vi "CLC_Gen3_L2_Manual_GUI.vi"() -> ()   [LabVIEW 2023, in "Clover_Cell.lvlib"]
uses:
  Clover_Cell.lvlib
  lib/Anritsu Signal Analyzer Series/Anritsu Signal Analyzer Series.lvlib
panel:
  in  "clear":bool
  out "Waveform Chart":dbl(graph)
  in  "Close":bool
  out "AvgTimes 2":i32=3
  out "Looping Times":i32
  out "error out":errorcluster
  in  "AvgTimes":i32=3
  in  "Start":bool
  in  "stop":bool
  in  "CenterFreq(GHz)":dbl=28.0
  in  "VISA resource name":refnum<visa-resource-name>="TCPIP0::192.168.100.230::inst0::INSTR"
  # "SA Record Tool ( Only )"
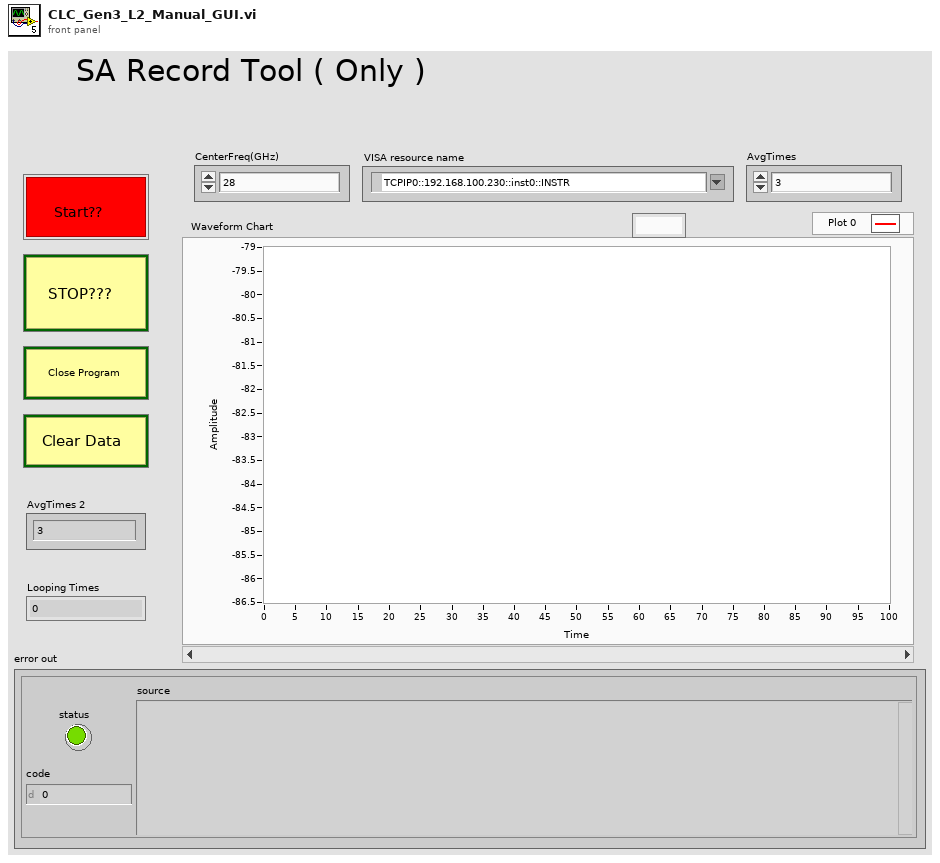
[diagram p1: front panel]
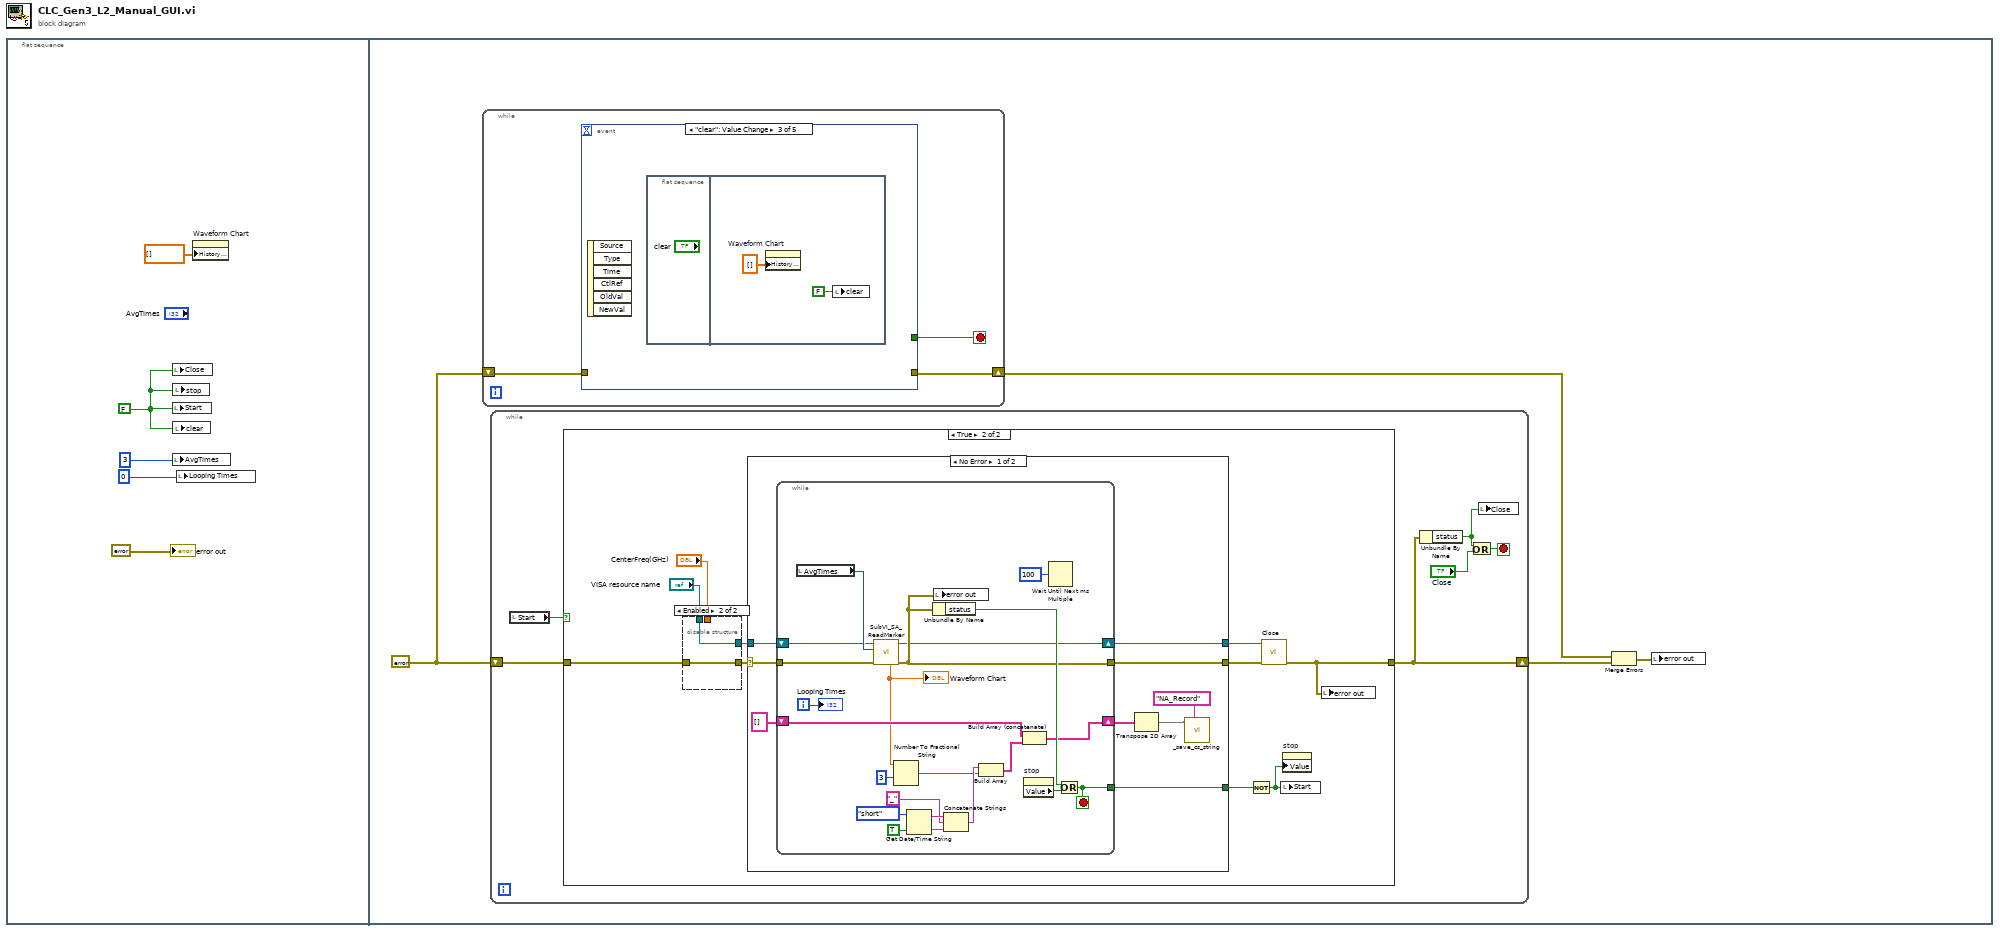
[diagram p0: block diagram]
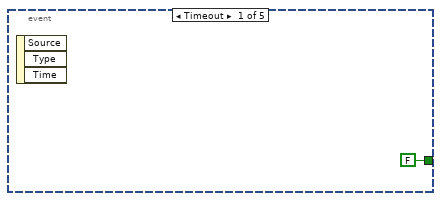
[diagram p2: hidden frame]
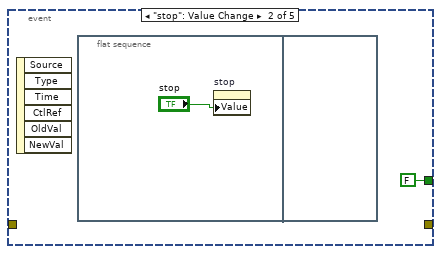
[diagram p3: hidden frame]
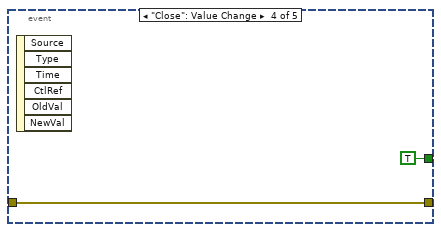
[diagram p4: hidden frame]
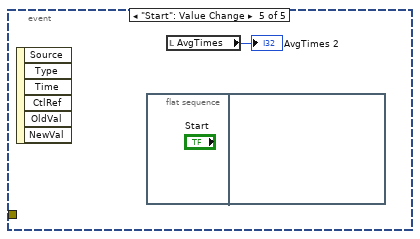
[diagram p5: hidden frame]
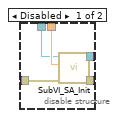
[diagram p7: hidden frame]
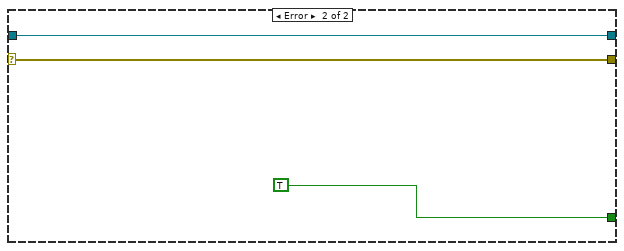
[diagram p8: hidden frame]
diagram:
  n1 = flat-sequence {
    frame #0 {
      w1 = FALSE ("Initialize")
      n2 = local write "Close"(w1) -> ()
      n3 = local write "Start"(w1) -> ()
      n4 = local write "AvgTimes"(3 ("AvgTimes")) -> ()
      n5 = local write "stop"(w1) -> ()
      n6 = local write "clear"(w1) -> ()
      n7 = local write "Looping Times"(0 ("Looping Times")) -> ()
      n8 = property on="Waveform Chart" class="WFChart (strict)"("History Data"=dbl[] []) -> ()  [unwired: 2 in, 2 out]
      "error out" <- errorcluster {"status"=FALSE, "code"=0, "source"=""} ("error in (no error)")
    }
    frame #1 {
      w9 = errorcluster {"status"=FALSE, "code"=0, "source"=""} ("error in (no error)")
      n9 = while {
        shift-right: [w10] -> w8
        shift-left: w9 -> [w11]
        stop <- w12 stop-if-true
        n10 = event shown="[2] \"clear\": Value Change" {
          selector: _ -> [_ _ _ _ _]
          dyn-events: _ -> [_ _ _ _ _]
          timeout: _ -> [_ _ _ _ _]
          tunnel: [FALSE ("stop") FALSE ("stop") _ TRUE ("stop") _] -> w12
          tunnel: w11 -> [_ _ _ w18 _]
          tunnel: [_ _ _ w18 _] -> w10
          event Timeout {
            n11 = event-data() -> ()  [unwired: 1 in, 3 out]
          }
          event "stop": Value Change {
            n12 = event-data() -> ()  [unwired: 1 in, 6 out]
            n13 = flat-sequence {
              frame #0 {
                n14 = property on="stop" class="Bool (strict)"("Value"="stop") -> ()  [unwired: 2 in, 2 out]
              }
              frame #1 {
              }
            }
          }
          event "clear": Value Change {
            n15 = event-data() -> ()  [unwired: 1 in, 6 out]
            n16 = flat-sequence {
              frame #0 {
              }
              frame #1 {
                n17 = property on="Waveform Chart" class="WFChart (strict)"("History Data"=dbl[] []) -> ()  [unwired: 2 in, 2 out]
                n18 = local write "clear"(FALSE ("clear")) -> ()
              }
            }
          }
          event "Close": Value Change {
            n19 = event-data() -> ()  [unwired: 1 in, 6 out]
          }
          event "Start": Value Change {
            n20 = event-data() -> ()  [unwired: 1 in, 6 out]
            n21 = flat-sequence {
              frame #0 {
              }
              frame #1 {
              }
            }
            n22 = local read "AvgTimes"() -> (→"AvgTimes 2":i32)
          }
        }
      }
      n23 = while {
        shift-right: [w24] -> w7
        shift-left: w9 -> [w25]
        stop <- w22 stop-if-true
        n24 = local read "Start"() -> (w26:bool)
        n25 = case shown="True" w26 {
          tunnel: w25 -> [w27 w31]
          tunnel: [w27 w33] -> w24
          frame False {
          }
          frame True {
            n26 = disable-structure shown="Enabled" {
              disable-tunnel: "CenterFreq(GHz)" -> [w42 _]
              disable-tunnel: w31 -> [w41 w44]
              disable-tunnel: "VISA resource name" -> [w40 w43]
              disable-tunnel: [w39 w43] -> w29
              disable-tunnel: [w38 w44] -> w28
              frame Disabled {
                n27 = call "SubVI_SA_Init.vi"("error in (no error)"=w41, "CenterFreq(GHz) 2"=w42, "VISA resource name"=w40) -> ("error out 2"=w38:errorcluster, "VISA resource name out"=w39:refnum<visa-resource-name>)  [unwired: 6 in, 1 out]
              }
              frame Enabled {
              }
            }
            n28 = case shown="No Error" w28 {
              selector: w28 -> [w49 w78]
              tunnel: [w53 TRUE] -> w37
              tunnel: [w52 w78] -> w35
              tunnel: [w51 w77] -> w34
              tunnel: w29 -> [w50 w77]
              frame No Error {
                n29 = while {
                  tunnel: [w72] -> w53
                  tunnel: [w69] -> w52
                  shift-right: [w68] -> w51
                  shift-left: w50 -> [w66]
                  tunnel: w49 -> [w67]
                  shift-right: [w55] -> w47
                  shift-left: string[][] [] -> [w56]
                  i -> [w74]
                  stop <- w72 stop-if-true
                  n30 = local read "AvgTimes"() -> (w70:i32)
                  n31 = call "SubVI_SA_ReadMarker.vi"("error in (no error)"=w67, "AvgTimes"=w70, "VISA resource name"=w66) -> ("error out"=w69:errorcluster, "VISA resource name out"=w68:refnum<visa-resource-name>, "Marker Power"=w54:dbl)  [unwired: 5 in, 1 out]
                  "Waveform Chart" <- w54
                  n32 = Number To Fractional String(number=w54, precision (6)=i16 3) -> (F-format string=w58:string)  [unwired: 2 in]
                  n33 = Get Date/Time String(date format (0)=enum16{"short", "long", "abbreviated"}."short", want seconds? (F)=TRUE) -> (date string=w64:string, time string=w63:string)  [unwired: 1 in]
                  n34 = Unbundle By Name(w69) -> ("status"=w75:bool)
                  n35 = local write "error out"(w69) -> ()
                  n36 = Concatenate Strings(w64, "_" ("string"), w63) -> (w59:string)
                  n37 = Build Array(w59, w58) -> (w57:string[])
                  n38 = Build Array (concatenate)(w56, w57) -> (w55:string[][])
                  n39 = property on="stop" class="Bool (strict)"() -> ("Value"=w71:bool)  [unwired: 2 in, 2 out]
                  n40 = Wait Until Next ms Multiple(millisecond multiple=u32 100) -> ()  [unwired: 1 out]
                  n41 = Or(x=w75, y=w71) -> (x .or. y?=w72:bool)
                  "Looping Times" <- w74
                }
                n42 = Transpose 2D Array(2D array=w47) -> (transposed array=w45:string[][])
                n43 = call "_save_cs_string.vi"("FileName"="NA_Record", "Array"=w45) -> ()  [unwired: 9 in, 1 out]
              }
              frame Error {
              }
            }
            n44 = Not(x=w37) -> (.not. x?=w36:bool)
            n45 = call "Close.vi"("error in (no error)"=w35, "VISA resource name"=w34) -> ("error out"=w33:errorcluster)  [unwired: 9 in]
            n46 = local write "Start"(w36) -> ()
            n47 = property on="stop" class="Bool (strict)"("Value"=w36) -> ()  [unwired: 2 in, 2 out]
            n48 = local write "error out"(w33) -> ()
          }
        }
        n49 = Unbundle By Name(w24) -> ("status"=w21:bool)
        n50 = Or(x=w21, y="Close") -> (x .or. y?=w22:bool)
        n51 = local write "Close"(w21) -> ()
      }
      n52 = Merge Errors(w8, w7) -> (w6:errorcluster)
      n53 = local write "error out"(w6) -> ()
    }
  }
